vi "SUB_SFCS_CHK_RFPI_IPEI_INFO.vi"(2 "InfoName":string, 3 "Stage":string, 4 "SN":string, 5 "URL":string) -> (0 "length":i32, 1 "output param":string)   [LabVIEW 2011]
uses:
  data/MCSDLL.dll
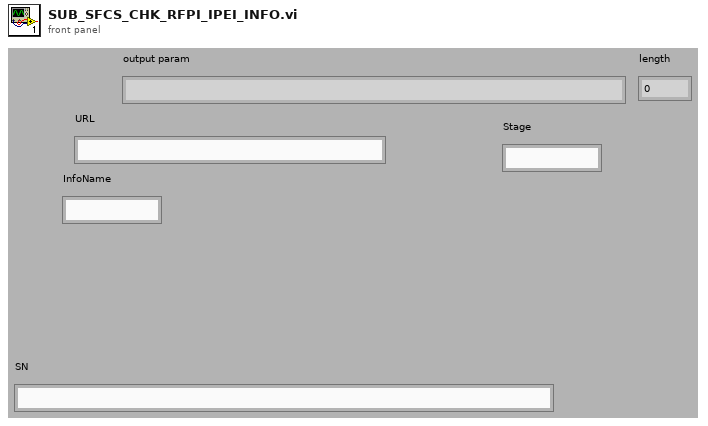
[diagram p1: front panel]
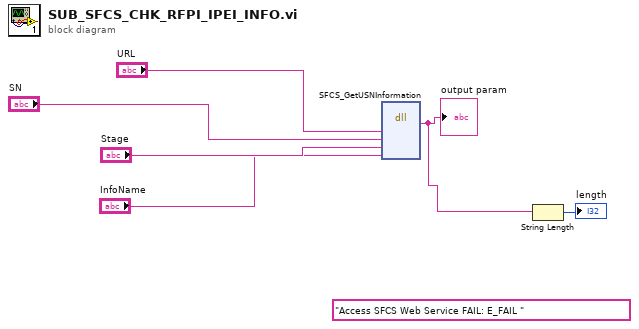
[diagram p0: block diagram]
diagram:
  (unwired) "Access SFCS Web Service FAIL: E_FAIL "
  n1 = dll-call lib="D:/S8300E_Project/data/MCSDLL.dll" fn="SFCS_GetUSNInformation"("URL"="URL", "SN"="SN", "Stage"="Stage", "InfoName"="InfoName") -> (w2:string)  [unwired: 7 in, 2 out]
  "output param" <- w2
  n2 = String Length(string=w2) -> (length=→"length":i32)
